vi "低层函数.vi"() -> ()   [LabVIEW 2018]
uses:
  <vilib>/userdefined/High Color/IMAQdx.ctl
  <vilib>/vision/driver/IMAQdx.llb/IMAQdx Acquisition Mode.ctl
  <vilib>/vision/driver/IMAQdx.llb/IMAQdx Buffer Number Mode.ctl
  <vilib>/vision/driver/NI_Vision_Acquisition_Software.lvlib
panel:
  out "error out":errorcluster
  out "Buffer Number Out":u32
  out "Image":T1(plugin-control)
  in  "error in":errorcluster
  in  "Session In":T2
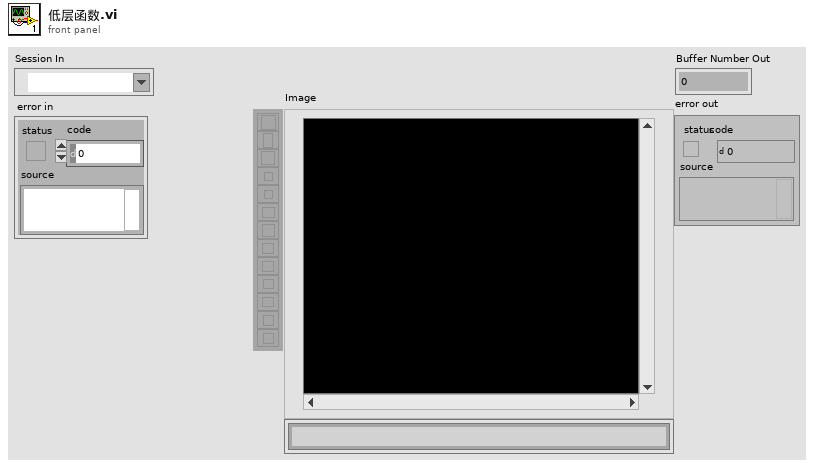
[diagram p1: front panel]
types:
  T1 = typedef "IMAQ Image.ctl" = refnum<image>
  T2 = typedef "IMAQdx.ctl" = refnum<k21>
  T3 = typedef "NI_Vision_Acquisition_Software.lvlib/IMAQdx Acquisition Mode.ctl" = enum32{"One Shot", "Continuous"}
  T4 = typedef "NI_Vision_Acquisition_Software.lvlib/IMAQdx Buffer Number Mode.ctl" = enum32{"Next", "Last", "Buffer Number", "Every", "Last New"}
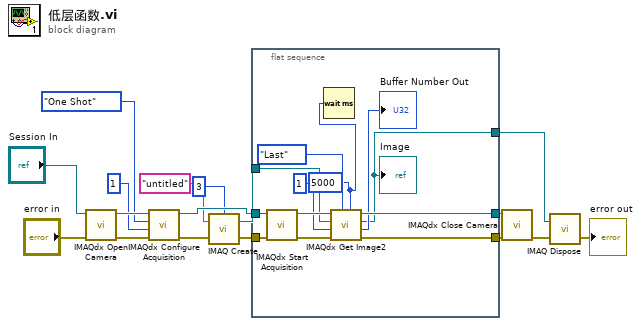
[diagram p0: block diagram]
diagram:
  n1 = call <vilib>:"IMAQdx Open Camera.vi"("error in"="error in", "Session In"="Session In") -> ("error out"=w12:errorcluster, "Session Out"=w16:T2)  [unwired: 8 in]
  n2 = call <vilib>:"IMAQdx Configure Acquisition.vi"("error in"=w12, "Number of Buffers"=u32 1, "Continuous?"=IMAQdx_Acquisition_Mode."One Shot", "Session In"=w16) -> ("error out"=w17:errorcluster, "Session Out"=w11:T2)  [unwired: 6 in]
  n3 = call "IMAQ Create"("Border Size"=3, "Image Name"="untitled", "error in (no error)"=w17) -> ("New Image"=w9:T1, "error out"=w8:errorcluster)  [unwired: 2 in]
  n4 = flat-sequence {
    tunnel: w11 -> [w27]
    tunnel: w9 -> [w26]
    tunnel: w8 -> [w25]
    tunnel: [w22] -> w6
    tunnel: [w21] -> w5
    tunnel: [w19] -> w3
    frame #0 {
      w18 = 5000 ("Timeout (ms)")
      n5 = call <vilib>:"IMAQdx Start Acquisition.vi"("error in"=w25, "Session In"=w27) -> ("error out"=w28:errorcluster, "Session Out"=w29:T2)  [unwired: 8 in]
      n6 = Wait (ms)(milliseconds to wait=w18) -> ()  [unwired: 1 out]
      n7 = call <vilib>:"IMAQdx Get Image2.vi"("Timeout (ms)"=w18, "Buffer Number Mode (Next)"=IMAQdx_Buffer_Number_Mode."Last", "error in"=w28, "Buffer Number In"=u32 1, "Image In"=w26, "Session In"=w29) -> ("error out"=w21:errorcluster, "Buffer Number Out"=→"Buffer Number Out":u32, "Image Out"=w19:T1, "Session Out"=w22:T2)  [unwired: 2 in]
      "Image" <- w19
    }
  }
  n8 = call <vilib>:"IMAQdx Close Camera.vi"("error in"=w5, "Session In"=w6) -> ("error out"=w4:errorcluster)  [unwired: 9 in]
  n9 = call "IMAQ Dispose"("Image"=w3, "error in (no error)"=w4) -> ("error out"=→"error out":errorcluster)  [unwired: 4 in]
